vi "Live Imaging Window.vi"() -> ()   [LabVIEW 2017]
uses:
  Typedefs/Channel Selector.ctl
  SubVIs/Typedefs/Live window-ctrl refs.ctl
  Typedefs/Image display ref.ctl
  Typedefs/Left-Right enum.ctl
  Global Variables/General Globals.vi
  Globals/gl_Windows Ctrl refs.vi
panel:
  in  "Boolean":bool=TRUE
  in  "Pal":u32(ring) items=["Grayscale", "Binary", "Gradient", "Rainbow", "Temperature", "User Defined"]
  out "Running":bool
  out "Stop (ind)":bool
  in  "Snapshot Mode":bool
  out "Images received":i32
  out "Acq rate ind (Hz)":dbl format="Acquisition frame rate: %.1f fps"
  out "Refresh rate ind (Hz)":i32 format="Graph refresh rate: %.0f fps"
  in  "Right image intensity":cluster{i16, i16}(slide)={0, 2048} scale=0.0..4095.0
  in  "Right Image Palette":enum16{"Gray", "Red", "Green"}(ring) caption="Palette"
  in  "Right Channel":T1=enum."Green Channel"
  in  "Left image intensity":cluster{i16, i16}(slide)={0, 2048} scale=0.0..4095.0
  in  "Left Image Palette":enum16{"Gray", "Red", "Green"}(ring) caption="Palette"
  in  "Left Channel":T1
  in  "Sim":bool
  out "Right Image":T2(plugin-control)
  in  "Snapshot":bool
  out "Left Image":T2(plugin-control)
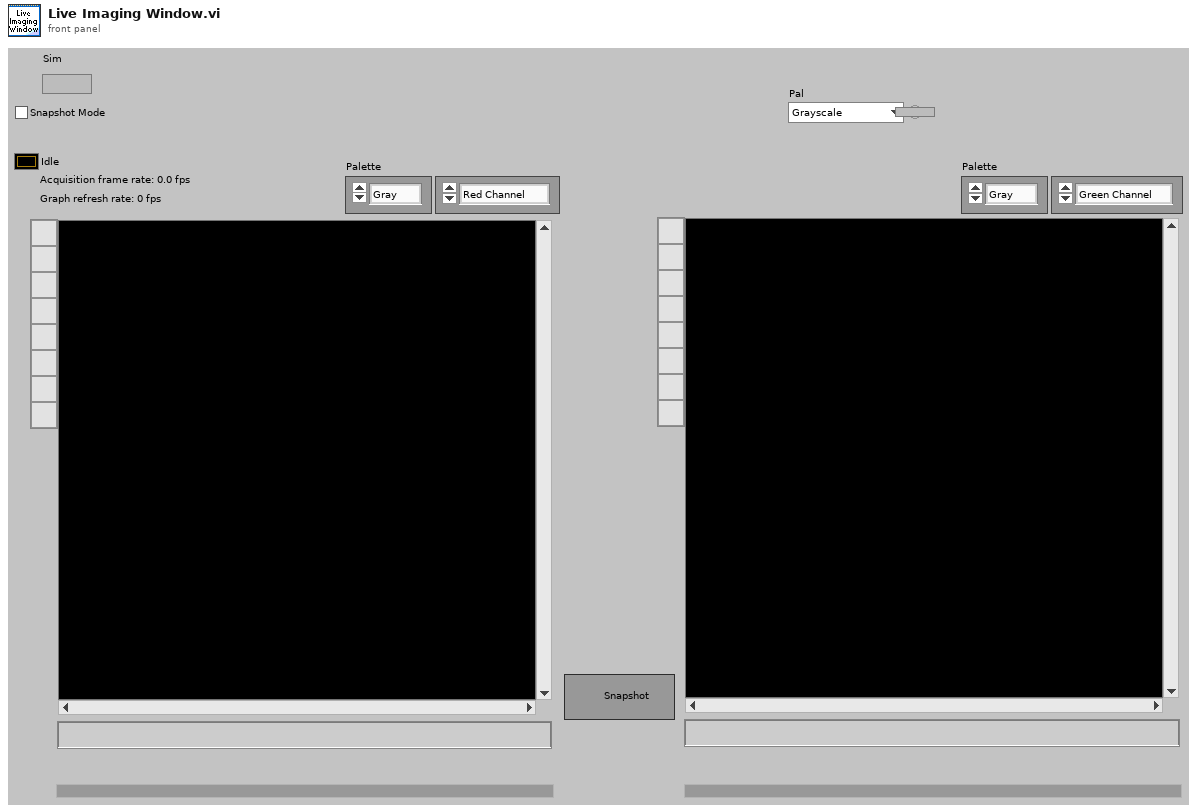
[diagram p1: front panel]
types:
  T1 = typedef "Channel Selector.ctl" = enum16{"Red Channel", "Green Channel", "Blended"}
  T2 = typedef "IMAQ Image.ctl" = refnum<image>
  T3 = typedef "Live window-ctrl refs.ctl" = cluster{"This VI":refnum<vi>, "Pane":refnum<vi>, "Snapshot":refnum<vi>, "Left Image Palette":refnum<vi>, "Right Image Palette":refnum<vi>, "Left Channel":refnum<vi>, "Right Channel":refnum<vi>, "Left image intensity":refnum<vi>, "Right image intensity":refnum<vi>, "Left Image Display":T4, "Right Image Display":T4, "Refresh rate ind (Hz)":refnum<vi>, "Acq rate ind (Hz)":refnum<vi>, "Stop (ind)":refnum<vi>}
  T4 = typedef "Image display ref.ctl" = refnum<vi>
  T5 = typedef "Live graph data queue ref.ctl" = refnum<queue>
  T6 = typedef "Live imaging queue element.ctl" = cluster{"Red channel":T2, "Green channel":T2}
  T7 = typedef "Left-Right enum.ctl" = enum16{"Right", "Left"}
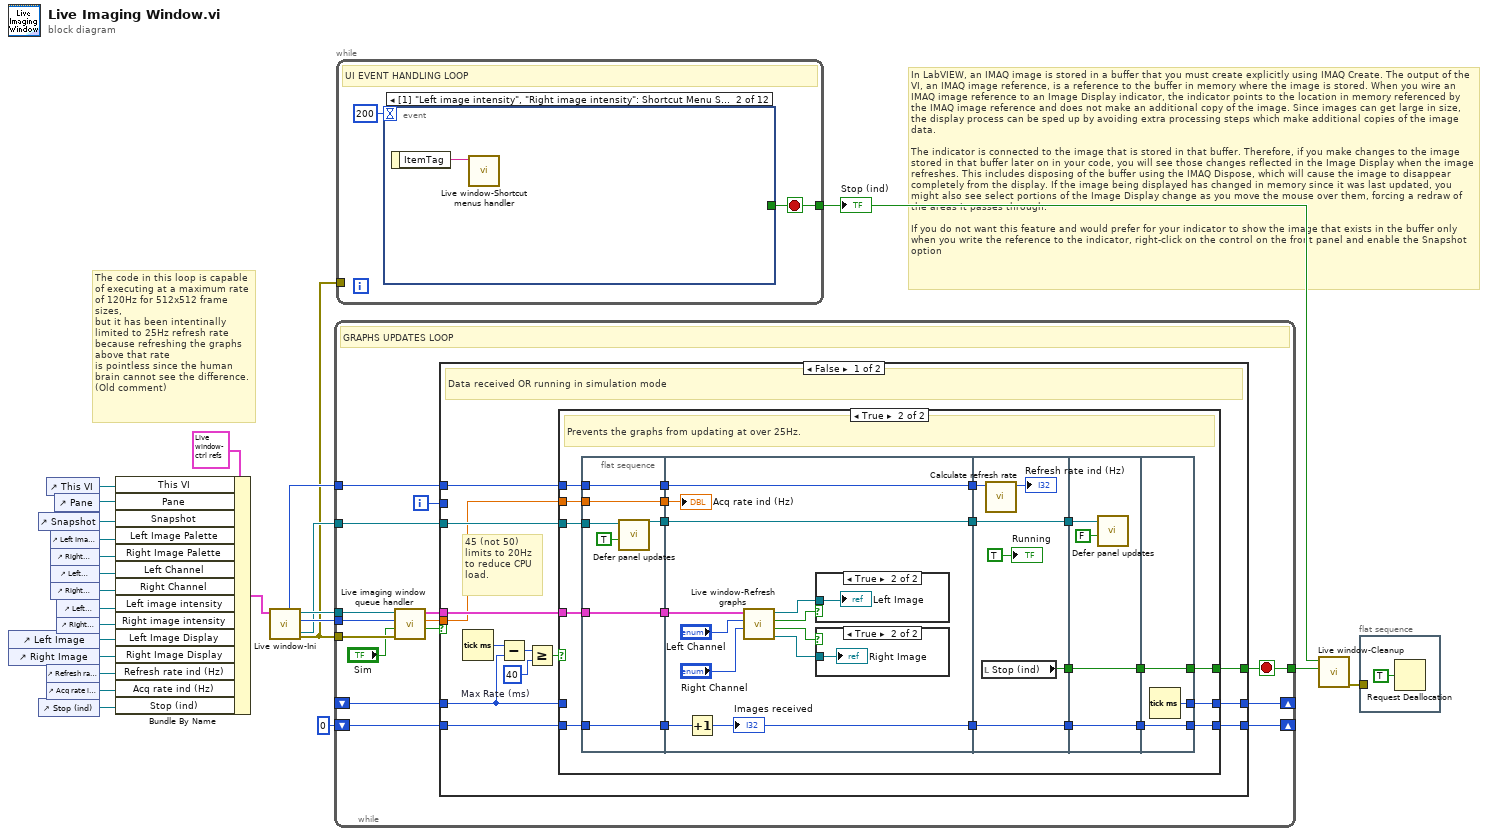
[diagram p0: block diagram]
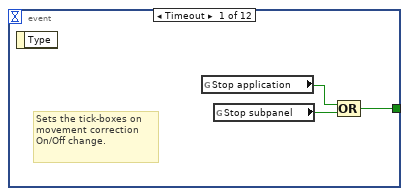
[diagram p2: hidden frame]
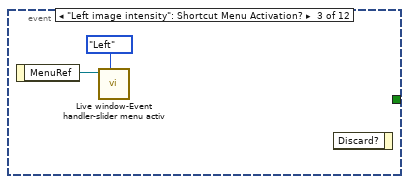
[diagram p3: hidden frame]
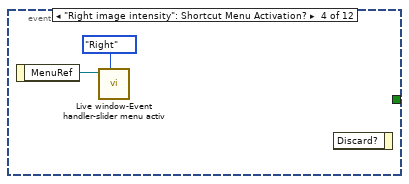
[diagram p4: hidden frame]
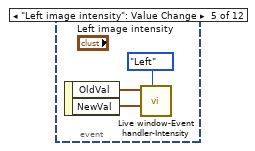
[diagram p5: hidden frame]
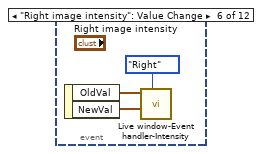
[diagram p6: hidden frame]
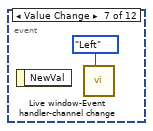
[diagram p7: hidden frame]
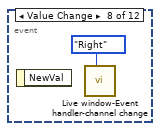
[diagram p8: hidden frame]
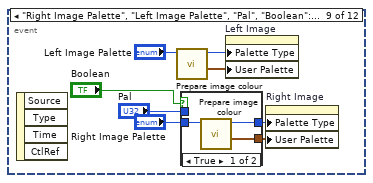
[diagram p9: hidden frame]
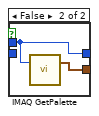
[diagram p10: hidden frame]
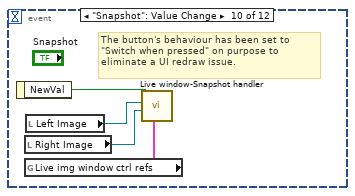
[diagram p11: hidden frame]
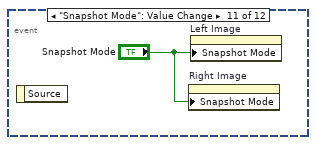
[diagram p12: hidden frame]
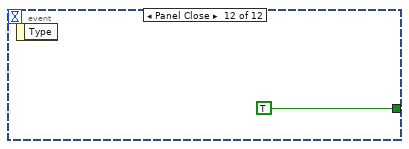
[diagram p13: hidden frame]
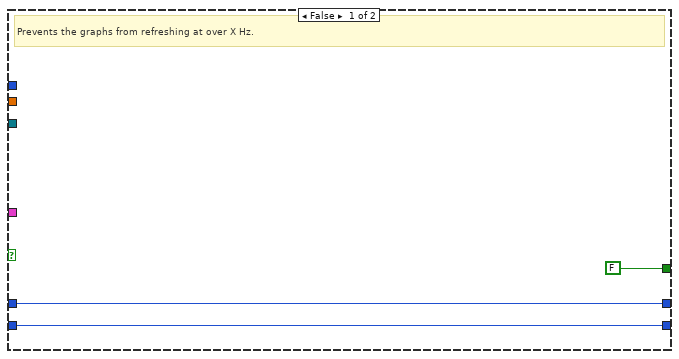
[diagram p14: hidden frame]
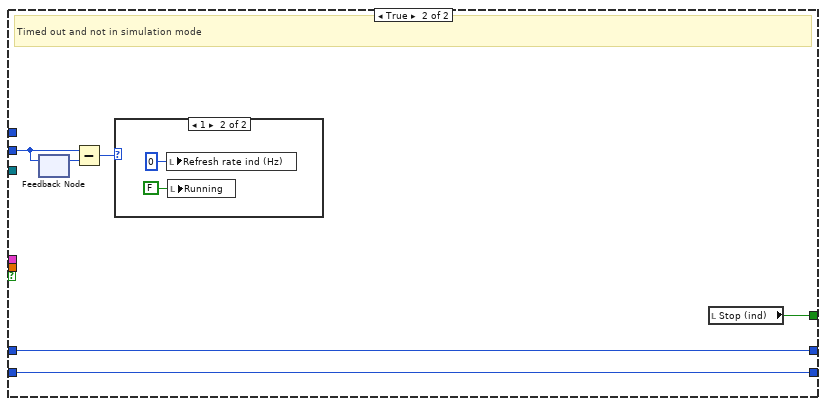
[diagram p17: hidden frame]
diagram:
  # "The code in this loop is capable of executing at a maximum rate of 120Hz for 512x512 frame sizes,\nbut it has been intentinally limited to 25Hz refresh rate because refreshing the graphs above that rate\nis pointless since the human brain cannot see the difference. (Old comment)"
  # "In LabVIEW, an IMAQ image is stored in a buffer that you must create explicitly using IMAQ Create. The output of the VI, an IMAQ image reference, is a reference to the buffer in memory where the image is stored. When you wire an IMAQ image reference to an Image Display indicator, the indicator points to the location in memory referenced by the IMAQ image reference and does not make an additional copy of the image. Since images can get large in size, the display process can be sped up by avoiding extra processing steps which make additional copies of the image data.\n\nThe indicator is connected to the image that is stored in that buffer. Therefore, if you make changes to the image stored in that buffer later on in your code, you will see those changes reflected in the Image Display when the image refreshes. This includes disposing of the buffer using the IMAQ Dispose, which will cause the image to disappear completely from the display. If the image being displayed has changed in memory since it was last updated, you might also see select portions of the Image Display change as you move the mouse over them, forcing a redraw of the areas it passes through.\n\nIf you do not want this feature and would prefer for your indicator to show the image that exists in the buffer only when you write the reference to the indicator, right-click on the control on the front panel and enable the Snapshot option"
  n1 = control-ref of="Left Image"() -> (w10:refnum<vi>)
  n2 = control-ref of="Right Image"() -> (w9:refnum<vi>)
  n3 = control-ref of="Snapshot"() -> (w13:refnum<vi>)
  n4 = control-ref of="Stop (ind)"() -> (w3:refnum<vi>)
  n5 = control-ref of="This VI"() -> (w15:refnum<vi>)
  n6 = control-ref of="Refresh rate ind (Hz)"() -> (w5:refnum<vi>)
  n7 = control-ref of="Acq rate ind (Hz)"() -> (w4:refnum<vi>)
  n8 = control-ref of="Left Image Palette"() -> (w21:refnum<vi>)
  n9 = control-ref of="Right Image Palette"() -> (w20:refnum<vi>)
  n10 = control-ref of="Left Channel"() -> (w19:refnum<vi>)
  n11 = control-ref of="Right Channel"() -> (w18:refnum<vi>)
  n12 = control-ref of="Pane"() -> (w7:refnum<vi>)
  n13 = control-ref of="Left image intensity"() -> (w17:refnum<vi>)
  n14 = control-ref of="Right image intensity"() -> (w16:refnum<vi>)
  n15 = Bundle By Name(cluster=T3 {"This VI"=refnum, "Pane"=refnum, "Snapshot"=refnum, "Left Image Palette"=refnum, "Right Image Palette"=refnum, "Left Channel"=refnum, "Right Channel"=refnum, "Left image intensity"=refnum, "Right image intensity"=refnum, "Left Image Display"=refnum, "Right Image Display"=refnum, "Refresh rate ind (Hz)"=refnum, "Acq rate ind (Hz)"=refnum, "Stop (ind)"=refnum} ("Live imaging window ctrl refs"), "This VI"=w15, "Pane"=w7, "Snapshot"=w13, "Left Image Palette"=w21, "Right Image Palette"=w20, "Left Channel"=w19, "Right Channel"=w18, "Left image intensity"=w17, "Right image intensity"=w16, "Left Image Display"=w10, "Right Image Display"=w9, "Refresh rate ind (Hz)"=w5, "Acq rate ind (Hz)"=w4, "Stop (ind)"=w3) -> (w11:T3)
  n16 = call "Live window-Ini.vi"("Live img window ctrl refs"=w11) -> ("error out"=w6:errorcluster, "Queue timeout"=w23:i32, "queue out"=w24:T5, "Front Panel"=w22:refnum<vi>, "Frame size"=w25:u16)  [unwired: 6 in]
  n17 = while {
    tunnel: w24 -> [w40]
    tunnel: w6 -> [w39]
    tunnel: w23 -> [w37]
    tunnel: [w27] -> w12
    shift-right: [w35] -> _
    shift-left: 0 -> [w31]
    tunnel: w25 -> [w34]
    shift-right: [w33] -> _
    shift-left: _ -> [w32]
    tunnel: w22 -> [w29]
    i -> [w26]
    stop <- w27 stop-if-true
    # "GRAPHS UPDATES LOOP"
    n18 = call "Live imaging window queue handler.vi"("error in (no error)"=w39, "Sim"="Sim", "timeout in ms"=w37, "Queue in"=w40) -> ("timed out?"=w30:bool, "Frame rate (Hz)"=w28:dbl, "Element to queue"=w38:T6)  [unwired: 5 in]
    n19 = case shown="False" w30 {
      tunnel: w38 -> [w53 _]
      tunnel: [w52 w117] -> w35
      tunnel: w31 -> [w45 w117]
      tunnel: w34 -> [w46 _]
      tunnel: [w51 w116] -> w33
      tunnel: w32 -> [w48 w116]
      tunnel: w29 -> [w44 _]
      tunnel: w28 -> [w43 _]
      tunnel: [w42 w115] -> w27
      tunnel: w26 -> [_ w113]
      frame False {
        w41 = u32 40  # Max Rate (ms)
        # "45 (not 50)\nlimits to 20Hz\nto reduce CPU\nload."
        # "Data received OR running in simulation mode"
        n20 = Tick Count (ms)() -> (millisecond timer value=w50:u32)
        n21 = Subtract(x=w50, y=w48) -> (x-y=w49:u32)
        n22 = Greater Or Equal?(x=w49, y=w41) -> (x >= y?=w47:bool)
        n23 = case shown="True" w47 {
          tunnel: w53 -> [_ w77]
          tunnel: [w56 w76] -> w52
          tunnel: [w55 w75] -> w51
          tunnel: w45 -> [w56 w74]
          tunnel: w48 -> [w55 _]
          tunnel: w46 -> [_ w73]
          tunnel: w44 -> [_ w72]
          tunnel: w43 -> [_ w66]
          tunnel: [FALSE w59] -> w42
          frame False {
            # "Prevents the graphs from refreshing at over X Hz."
          }
          frame True {
            # "Prevents the graphs from updating at over 25Hz."
            n24 = flat-sequence {
              tunnel: w66 -> [w81]
              tunnel: w72 -> [w80]
              tunnel: w73 -> [w82]
              tunnel: w77 -> [w83]
              tunnel: w74 -> [w84]
              tunnel: [w84] -> w65
              tunnel: [w83] -> w64
              tunnel: [w82] -> w63
              tunnel: [w79] -> w62
              tunnel: [w81] -> w61
              tunnel: [w90] -> w71
              tunnel: [w96] -> w69
              tunnel: [w88] -> w68
              tunnel: w65 -> [w91]
              tunnel: w64 -> [w89]
              tunnel: w63 -> [w96]
              tunnel: w62 -> [w88]
              tunnel: w61 -> [w87]
              tunnel: w71 -> [w104]
              tunnel: [w104] -> w70
              tunnel: w69 -> [w101]
              tunnel: w68 -> [w103]
              tunnel: [w103] -> w67
              tunnel: [w99] -> w57
              tunnel: w70 -> [w108]
              tunnel: w67 -> [w107]
              tunnel: [w108] -> w60
              tunnel: [w106] -> w58
              tunnel: w57 -> [w106]
              tunnel: [w110] -> w75
              tunnel: [w111] -> w76
              tunnel: w60 -> [w111]
              tunnel: [w109] -> w59
              tunnel: w58 -> [w109]
              frame #0 {
                n25 = call "Defer panel updates.vi"("Defer Panel Updates"=TRUE, "Panel in"=w80) -> ("Panel out"=w79:refnum<vi>)  [unwired: 9 in]
              }
              frame #1 {
                n26 = Increment(x=w91) -> (x+1=w90:i32)
                "Images received" <- w90
                n27 = call "Live window-Refresh graphs.vi"("Right Channel"="Right Channel", "Left Channel"="Left Channel", "Element to queue"=w89) -> ("Right image"=w94:T2, "Enable right image"=w92:bool, "Enable left image"=w93:bool, "Left image"=w95:T2)  [unwired: 5 in]
                n28 = case shown="True" w93 {
                  tunnel: w95 -> [_ w98]
                  frame False {
                  }
                  frame True {
                    "Left Image" <- w98
                  }
                }
                n29 = case shown="True" w92 {
                  tunnel: w94 -> [_ w97]
                  frame False {
                  }
                  frame True {
                    "Right Image" <- w97
                  }
                }
                "Acq rate ind (Hz)" <- w87
              }
              frame #2 {
                n30 = local read "Stop (ind)"() -> (w99:bool)
                n31 = call "Calculate refresh rate.vi"("Frame size"=w101) -> ("Refresh rate (Hz)"=→"Refresh rate ind (Hz)":i32)  [unwired: 9 in, 1 out]
                "Running" <- TRUE ("Running")
              }
              frame #3 {
                n32 = call "Defer panel updates.vi"("Defer Panel Updates"=FALSE, "Panel in"=w107) -> ()  [unwired: 9 in, 1 out]
              }
              frame #4 {
                n33 = Tick Count (ms)() -> (millisecond timer value=w110:u32)
              }
            }
          }
        }
      }
      frame True {
        # "Timed out and not in simulation mode"
        n34 = feedback-in #1(w113) -> ()
        n35 = feedback #1() -> (w114:i32)  [unwired: 1 in]
        n36 = Subtract(x=w113, y=w114) -> (x-y=w112:i32)
        n37 = case shown="1" w112 {
          frame Default {
          }
          frame 1 {
            n38 = local write "Refresh rate ind (Hz)"(0 ("Refresh rate ind (Hz)")) -> ()
            n39 = local write "Running"(FALSE ("Running")) -> ()
          }
        }
        n40 = local read "Stop (ind)"() -> (w115:bool)
      }
    }
  }
  n41 = while {
    tunnel: [w120] -> w1
    tunnel: w6 -> [_]
    stop <- w120 stop-if-true
    # "UI EVENT HANDLING LOOP"
    n42 = event shown="[1] \"Left image intensity\", \"Right image intensity\": Shortcut Menu Selection (User)" {
      selector: _ -> [_ _ _ _ _ _ _ _ _ _ _ _]
      dyn-events: _ -> [_ _ _ _ _ _ _ _ _ _ _ _]
      timeout: 200 -> [_ _ _ _ _ _ _ _ _ _ _ _]
      tunnel: [w122 _ _ _ _ _ _ _ _ _ _ TRUE] -> w120
      event Timeout {
        # "Sets the tick-boxes on movement correction On/Off change."
        n43 = event-data() -> ()  [unwired: 1 in, 1 out]
        n44 = global read "General Globals.vi" "Stop application"() -> (w123:bool)
        n45 = global read "General Globals.vi" "Stop subpanel"() -> (w124:bool)
        n46 = Compound Arithmetic op=OR(w123, w124) -> (w122:bool)
      }
      event "Left image intensity", "Right image intensity": Shortcut Menu Selection (User) {
        n47 = event-data() -> ("ItemTag"=w125:string)  [unwired: 1 in]
        n48 = call "Live window-Shortcut menus handler.vi"("ItemTag"=w125) -> ()  [unwired: 11 in]
      }
      event "Left image intensity": Shortcut Menu Activation? {
        n49 = event-data() -> ("MenuRef"=w127:refnum<k9>)  [unwired: 1 in]
        n50 = call "Live window-Event handler-slider menu activ.vi"("Left/Right"=Left-Right_enum."Left", "Image intensity slider Menu"=w127) -> ()  [unwired: 10 in]
        n51 = event-data() -> ()  [unwired: 2 in, 1 out]
      }
      event "Right image intensity": Shortcut Menu Activation? {
        n52 = event-data() -> ("MenuRef"=w128:refnum<k9>)  [unwired: 1 in]
        n53 = call "Live window-Event handler-slider menu activ.vi"("Left/Right"=Left-Right_enum."Right", "Image intensity slider Menu"=w128) -> ()  [unwired: 10 in]
        n54 = event-data() -> ()  [unwired: 2 in, 1 out]
      }
      event "Left image intensity": Value Change {
        n55 = event-data() -> ("OldVal"=w132:cluster{i16, i16}, "NewVal"=w131:cluster{i16, i16})  [unwired: 1 in]
        n56 = call "Live window-Event handler-Intensity.vi"("Which image display?"=Left-Right_enum."Left", "NewVal"=w131, "OldVal"=w132) -> ()  [unwired: 9 in]
      }
      event "Right image intensity": Value Change {
        n57 = event-data() -> ("OldVal"=w134:cluster{i16, i16}, "NewVal"=w135:cluster{i16, i16})  [unwired: 1 in]
        n58 = call "Live window-Event handler-Intensity.vi"("Which image display?"=Left-Right_enum."Right", "NewVal"=w135, "OldVal"=w134) -> ()  [unwired: 9 in]
      }
      event Value Change {
        n59 = event-data() -> ()  [unwired: 1 in, 1 out]
        n60 = call "Live window-Event handler-channel change.vi"("Left/Right"=Left-Right_enum."Left") -> ()  [unwired: 10 in, 1 out]
      }
      event Value Change {
        n61 = event-data() -> ()  [unwired: 1 in, 1 out]
        n62 = call "Live window-Event handler-channel change.vi"("Left/Right"=Left-Right_enum."Right") -> ()  [unwired: 10 in, 1 out]
      }
      event "Right Image Palette", "Left Image Palette", "Pal", "Boolean": Value Change {
        n63 = event-data() -> ()  [unwired: 1 in, 4 out]
        n64 = call "Prepare image colour.vi"("Left Image Palette"="Left Image Palette") -> ("Color Palette"=w143:cluster{"Red":u8, "Green":u8, "Blue":u8}[], "Palette Type"=w145:u32)  [unwired: 8 in, 1 out]
        n65 = case shown="True" "Boolean" {
          tunnel: [w148 w150] -> w142
          tunnel: "Right Image Palette" -> [w147 _]
          tunnel: [w146 w149] -> w140
          tunnel: "Pal" -> [_ w149]
          frame True {
            n66 = call "Prepare image colour.vi"("Left Image Palette"=w147) -> ("Color Palette"=w148:cluster{"Red":u8, "Green":u8, "Blue":u8}[], "Palette Type"=w146:u32)  [unwired: 8 in, 1 out]
          }
          frame False {
            n67 = call "IMAQ GetPalette"("Palette Number (gray)"=w149) -> ("Color Palette"=w150:cluster{"Red":u8, "Green":u8, "Blue":u8}[])  [unwired: 4 in, 1 out]
          }
        }
        n68 = property on="Left Image" class="ImageControl"("Palette Type"=w145, "User Palette"=w143) -> ()  [unwired: 2 in, 2 out]
        n69 = property on="Right Image" class="ImageControl"("Palette Type"=w140, "User Palette"=w142) -> ()  [unwired: 2 in, 2 out]
      }
      event "Snapshot": Value Change {
        # "The button's behaviour has been set to \"Switch when pressed\" on purpose to eliminate a UI redraw issue."
        n70 = event-data() -> ("NewVal"=w154:bool)  [unwired: 1 in]
        n71 = local read "Right Image"() -> (w152:T2)
        n72 = global read "gl_Windows Ctrl refs.vi" "Live img window ctrl refs"() -> (w151:T3)
        n73 = local read "Left Image"() -> (w153:T2)
        n74 = call "Live window-Snapshot handler.vi"("Window ctrl refs"=w151, "Right image"=w152, "Left image"=w153, "Snapshot:NewVal"=w154) -> ()  [unwired: 8 in]
      }
      event "Snapshot Mode": Value Change {
        n75 = event-data() -> ()  [unwired: 1 in, 1 out]
        n76 = property on="Right Image" class="ImageControl"("Snapshot Mode"="Snapshot Mode") -> ()  [unwired: 2 in, 2 out]
        n77 = property on="Left Image" class="ImageControl"("Snapshot Mode"="Snapshot Mode") -> ()  [unwired: 2 in, 2 out]
      }
      event Panel Close {
        n78 = event-data() -> ()  [unwired: 1 in, 1 out]
      }
    }
  }
  "Stop (ind)" <- w1
  n79 = call "Live window-Cleanup.vi"("Stop"=w12, "Boolean"=w1) -> ("error out"=w2:errorcluster)  [unwired: 9 in]
  n80 = flat-sequence {
    tunnel: w2 -> [_]
    frame #0 {
      n81 = Request Deallocation(TRUE ("flag")) -> ()
    }
  }
